vi "Manager QueryErrors.vi"(6 "contextId":T1, 8 "error in":errorcluster, 9 "timeout (ms)":i32=-1, 10 "Request Data":T5, 11 "gRPC ID":T1) -> (0 "error out":errorcluster, 2 "Response Data":T2, 3 "gRPC ID out":T1)   [LabVIEW 2021, in "CIF_Manager_client.lvlib"]
uses:
  CIF_Manager_client.lvlib
  <vilib>/gRPC/LabVIEW gRPC Library/Shared/grpcId.ctl
  RPC Messages/cif_manager_QueryErrorsRequest.ctl
  RPC Messages/cif_manager_QuerySettings.ctl
  RPC Messages/cif_manager_QueryErrorsResponse.ctl
  RPC Messages/cif_manager_ErrorInfoList.ctl
  RPC Messages/cif_manager_ErrorInfo.ctl
  RPC Messages/cif_manager_QueryErrorsResponse_Flat.ctl
  RPC Messages/cif_manager_ErrorInfoList_Flat.ctl
  RPC Messages/cif_manager_ErrorInfo_Flat.ctl
  14035477-4c25-4107-8ed5-d0c4ef420ce5.vi
  RPC Messages/RichToFlatcif_manager_QuerySettings.vi
  <vilib>/gRPC/LabVIEW gRPC Library/Shared/TranslateGrpcError.vi
  <vilib>/gRPC/LabVIEW gRPC Library/Shared/Wait On Occurrence.vi
  RPC Messages/FlatToRichcif_manager_ErrorInfoList.vi
  <vilib>/gRPC/LabVIEW gRPC Library/Shared/Is Feature Enabled.vi
  RPC Messages/FlatToRichcif_manager_ErrorInfo.vi
  <vilib>/gRPC/LabVIEW gRPC Library/Server API/Server/Get Server DLL Path.vi
  <vilib>/Utility/error.llb/Error Cluster From Error Code.vi
  <vilib>/gRPC/LabVIEW gRPC Library/grpc-lvsupport-release.lvlib
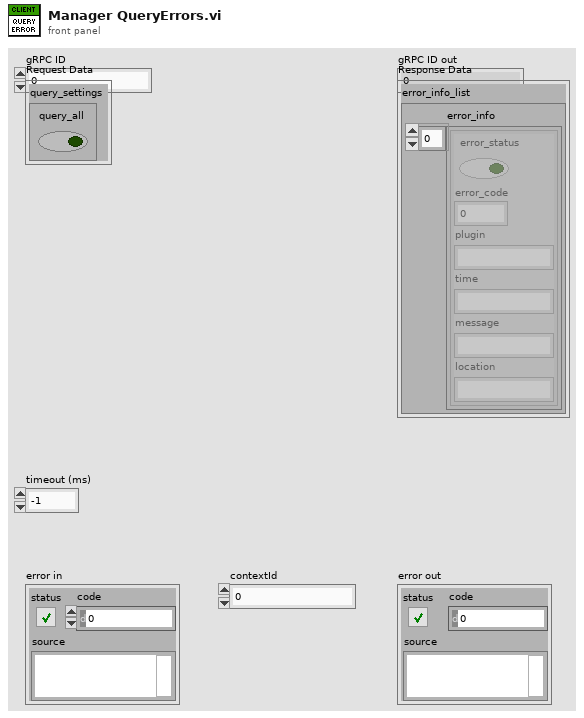
[diagram p1: front panel]
types:
  T1 = typedef "grpc-lvsupport-release.lvlib/grpcId.ctl" = u64
  T2 = typedef "CIF_Manager_client.lvlib/cif_manager_QueryErrorsResponse.ctl" = cluster{"error_info_list":T3}
  T3 = typedef "CIF_Manager_client.lvlib/cif_manager_ErrorInfoList.ctl" = cluster{"error_info":T4[]}
  T4 = typedef "CIF_Manager_client.lvlib/cif_manager_ErrorInfo.ctl" = cluster{"error_status":bool, "error_code":i32, "plugin":string, "time":string, "message":string, "location":string}
  T5 = typedef "CIF_Manager_client.lvlib/cif_manager_QueryErrorsRequest.ctl" = cluster{"query_settings":T6}
  T6 = typedef "CIF_Manager_client.lvlib/cif_manager_QuerySettings.ctl" = cluster{"query_all":bool}
  T7 = typedef "CIF_Manager_client.lvlib/cif_manager_QueryErrorsResponse_Flat.ctl" = cluster{"error_info_list":T8}
  T8 = typedef "CIF_Manager_client.lvlib/cif_manager_ErrorInfoList_Flat.ctl" = cluster{"error_info":T9[]}
  T9 = typedef "CIF_Manager_client.lvlib/cif_manager_ErrorInfo_Flat.ctl" = cluster{"error_status":bool, "error_code":i32, "plugin":string, "time":string, "message":string, "location":string}
  T10 = typedef "CIF_Manager_client.lvlib/cif_manager_QueryErrorsRequest_Flat.ctl" = cluster{"query_settings":T11}
  T11 = typedef "CIF_Manager_client.lvlib/cif_manager_QuerySettings_Flat.ctl" = cluster{"query_all":bool}
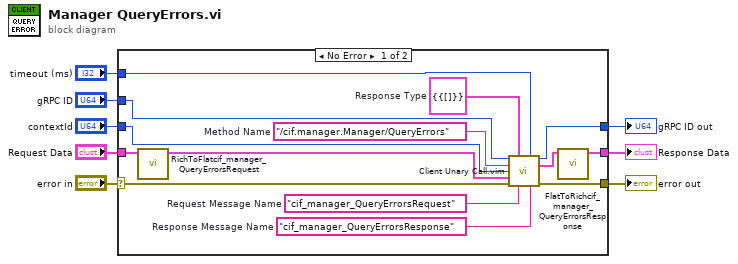
[diagram p0: block diagram]
diagram:
  n1 = case shown="No Error" "error in" {
    selector: "error in" -> [w18 w23]
    tunnel: [w17 w23] -> w7
    tunnel: "gRPC ID" -> [w16 w24]
    tunnel: [w15 w24] -> w5
    tunnel: "Request Data" -> [w12 _]
    tunnel: [w9 _] -> w3
    tunnel: "timeout (ms)" -> [w14 _]
    tunnel: "contextId" -> [w13 _]
    frame No Error {
      w19 = "cif_manager_QueryErrorsResponse"  # Response Message Name
      w20 = "cif_manager_QueryErrorsRequest"  # Request Message Name
      w21 = T7 {"error_info_list"={"error_info"=[]}}  # Response Type
      w22 = "/cif.manager.Manager/QueryErrors"  # Method Name
      n2 = call "RichToFlatcif_manager_QueryErrorsRequest.vi"("InputCluster"=w12) -> ("OutputCluster"=w11:T10)  [unwired: 10 in]
      n3 = call "Client Unary Call.vim"("ClientID in"=w16, "Response Type"=w21, "timeout (ms)"=w14, "Method Name"=w22, "contextId"=w13, "Request Data"=w11, "error in"=w18, "Request Message Name"=w20, "Response Message Name"=w19) -> ("ClientID out"=w15:u64, "Response Data"=w10:T7, "error out"=w17:errorcluster)  [unwired: 4 in]
      n4 = call "FlatToRichcif_manager_QueryErrorsResponse.vi"("InputCluster"=w10) -> ("OutputCluster"=w9:T2)  [unwired: 10 in]
    }
    frame Error {
    }
  }
  "error out" <- w7
  "gRPC ID out" <- w5
  "Response Data" <- w3
